vi "Check if Measurement Ready.vi"(8 "error in (no error)":errorcluster) -> (0 "error out":errorcluster)   [LabVIEW 2019]
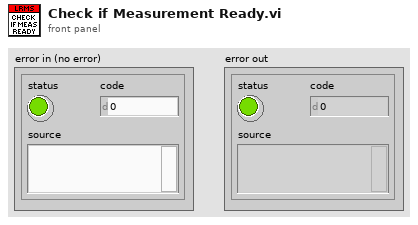
[diagram p1: front panel]
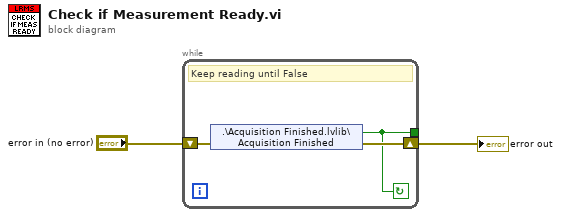
[diagram p0: block diagram]
diagram:
  n1 = while {
    shift-right: [w4] -> w1
    shift-left: "error in (no error)" -> [w5]
    tunnel: [w3] -> _
    stop <- w3 continue-if-true
    # "Keep reading until False"
    n2 = shared-variable ".\\Acquisition Finished.lvlib\\Acquisition Finished"(error in=w5) -> (w3:bool, error out=w4:errorcluster)
  }
  "error out" <- w1
